vi "Sync In (I2S).vi"(8 "receive":bool, 9 "prev transfer done":bool, 10 "sync in":bool) -> (0 "latch config":bool, 1 "force output":bool, 2 "start read":bool)   [LabVIEW 2013, in "I2S-TDM.lvlib"]
uses:
  I2S-TDM.lvlib
  Controls/i2s sync states.ctl
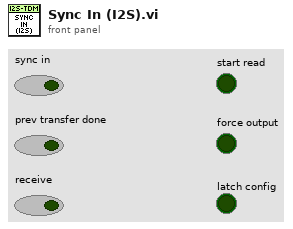
[diagram p1: front panel]
types:
  T1 = typedef "I2S-TDM.lvlib/i2s sync states.ctl" = enum16{"idle", "first word", "second word"}
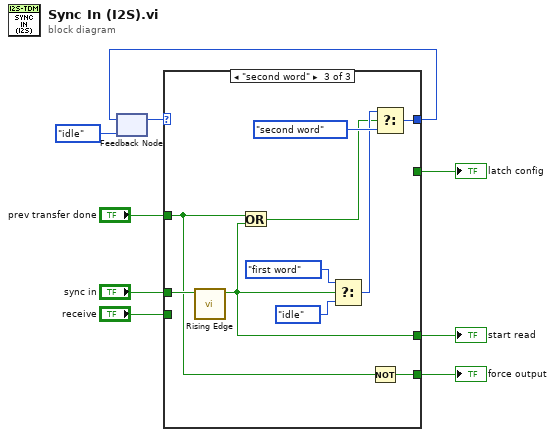
[diagram p0: block diagram]
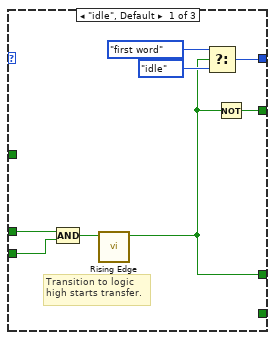
[diagram p2: hidden frame]
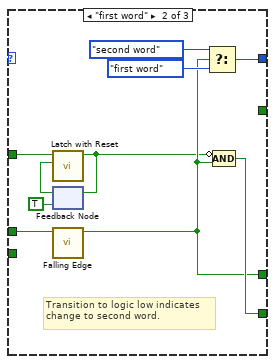
[diagram p3: hidden frame]
diagram:
  n1 = feedback #1(i2s_sync_states."idle" ("sync state")) -> (w9:T1)
  n2 = case shown="\"second word\"" w9 {
    tunnel: [w17 w25 w36] -> w4
    tunnel: [w10 w21 w30] -> w7
    tunnel: [w16 _ _] -> w8
    tunnel: [_ w22 w28] -> w6
    tunnel: "prev transfer done" -> [_ w23 w29]
    tunnel: "sync in" -> [w15 w24 w35]
    tunnel: "receive" -> [w11 _ _]
    frame "idle", Default {
      # "Transition to logic high starts transfer."
      n3 = Compound Arithmetic op=AND(w15, w11) -> (w14:bool)
      n4 = call "Rising Edge.vi"("signal in"=w14) -> ("rising edge?"=w10:bool)  [unwired: 10 in]
      n5 = Select(t=i2s_sync_states."first word" ("sync state"), s=w10, f=i2s_sync_states."idle" ("sync state")) -> (s? t:f=w17:T1)
      n6 = Not(x=w10) -> (.not. x?=w16:bool)
    }
    frame "first word" {
      # "Transition to logic low indicates change to second word."
      n7 = feedback #2(TRUE ("latched signal")) -> (w19:bool)
      n8 = call "Latch with Reset.vi"("reset"=w19, "signal"=w23) -> ("latched signal"=w20:bool)  [unwired: 9 in]
      n9 = feedback-in #2(w20) -> ()
      n10 = call "Falling Edge.vi"("signal in"=w24) -> ("falling edge?"=w21:bool)  [unwired: 10 in]
      n11 = Select(t=i2s_sync_states."second word" ("sync state"), s=w21, f=i2s_sync_states."first word" ("sync state")) -> (s? t:f=w25:T1)
      n12 = Compound Arithmetic op=AND(invert w20, w21) -> (w22:bool)
    }
    frame "second word" {
      n13 = call "Rising Edge.vi"("signal in"=w35) -> ("rising edge?"=w30:bool)  [unwired: 10 in]
      n14 = Or(x=w29, y=w30) -> (x .or. y?=w31:bool)
      n15 = Select(t=i2s_sync_states."first word" ("sync state"), s=w30, f=i2s_sync_states."idle" ("sync state")) -> (s? t:f=w32:T1)
      n16 = Not(x=w29) -> (.not. x?=w28:bool)
      n17 = Select(t=w32, s=w31, f=i2s_sync_states."second word" ("sync state")) -> (s? t:f=w36:T1)
    }
  }
  "start read" <- w7
  "latch config" <- w8
  "force output" <- w6
  n18 = feedback-in #1(w4) -> ()
